vi "Periodic Tasks.vi"(8 "error in":errorcluster) -> ()   [LabVIEW 2015]
doc: "This VI runs in parallel to other tasks. It can contain as many user-defined periodic loops as you need. These can carry out PID or other sorts of timed response."
uses:
  sprocket/src/Refname/Refname Enum (Actuator).ctl
  sprocket/src/Action/Action Name.ctl
  <vilib>/Rock Robotics/SystemInterfaces/Utilities/FPGA_UtilitiesLED Source.ctl
  <vilib>/Rock Robotics/SystemInterfaces/Utilities/FPGA_UtilitiesLED State.ctl
  <vilib>/Rock Robotics/WPI/Compressor/WPI_CompressorGetSetRefNum.vi
  <vilib>/Rock Robotics/WPI/RobotDrive/WPI_RobotDriveGetSetRefNum.vi
  Robot Global Data.vi
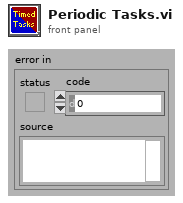
[diagram p1: front panel]
types:
  T1 = typedef "Refname Enum (Actuator).ctl" = enum16{"Drive Motors"}
  T2 = typedef "Action.ctl" = cluster{"Name":T3, "Priority":i32, "Data":variant}
  T3 = typedef "Action Name.ctl" = enum16{"No Action", "Drive Left", "Drive Right"}
  T4 = typedef "FPGA_UtilitiesLED State.ctl" = enum16{"Off", "On", "Toggle"}
  T5 = typedef "FPGA_UtilitiesLED Source.ctl" = enum16{"User LED", "FPGA LED"}
  T6 = typedef "WPI_CompressorDevRef.ctl" = cluster{"DevStatus":errorcluster, "DigitalInputDevRef":T7, "RelayDevRef":T10}
  T7 = typedef "WPI_DigitalInputDevRef.ctl" = cluster{"DevStatus":errorcluster, "DIO Channel":T8, "Digital Module":T9}
  T8 = typedef "FPGA_DIOChannel.ctl" = enum8{"DIO 1", "DIO 2", "DIO 3", "DIO 4", "DIO 5", "DIO 6", "DIO 7", "DIO 8", "DIO 9", "DIO 10", "DIO 11", "DIO 12", "DIO 13", "DIO 14", "Invalid"}
  T9 = typedef "FPGA_TypedefDigitalModule.ctl" = enum16{"Digital Module 1", "Digital Module 2"}
  T10 = typedef "WPI_RelayDevRef.ctl" = cluster{"DevStatus":errorcluster, "Relay Channel":T11, "Digital Module":T9, "Relay Direction":T12}
  T11 = typedef "FPGA_DIORelayChannel.ctl" = enum8{"Relay 1", "Relay 2", "Relay 3", "Relay 4", "Relay 5", "Relay 6", "Relay 7", "Relay 8", "Invalid"}
  T12 = typedef "WPI_RelayDirection.ctl" = enum16{"Both directions", "Forward only", "Reverse only"}
  T13 = typedef "WPI_RobotDriveDevRef.ctl" = cluster{"DevStatus":errorcluster, "Motors[]":T14[], "Square Inputs":bool, "Max Output":dbl}
  T14 = typedef "WPI_MotorControlDeviceRef.ctl" = cluster{"DeviceStatus":errorcluster, "Type":enum16{"PWM", "CAN"}, "PWM":cluster{"Digital Module":T9, "PWM Channel":T15, "DeadBand":T16}, "CAN":cluster{"Device Number":u8, "Control Mode":T17, "Semaphore":T18, "Max Vout":dbl}, "Invert":bool, "TransformRef":T19, "InvTransformRef":T19}
  T15 = typedef "FPGA_DIOPWMChannel.ctl" = enum8{"PWM 1", "PWM 2", "PWM 3", "PWM 4", "PWM 5", "PWM 6", "PWM 7", "PWM 8", "PWM 9", "PWM 10", "Invalid"}
  T16 = typedef "WPI_PWMDeadband.ctl" = cluster{"Name":string, "maxPositivePwm":i32, "minPositivePwm":i32, "centerPwm":i32, "maxNegativePwm":i32, "minNegativePwm":i32, "angularRange":u16}
  T17 = typedef "WPI_CANJaguar_ControlMode.ctl" = enum8{"Percent VBus", "Current", "Speed", "Position", "Voltage"}
  T18 = typedef "Semaphore RefNum" = refnum<k1>
  T19 = typedef "WPI_PWMTransform_ConPane.ctl" = refnum<vi>
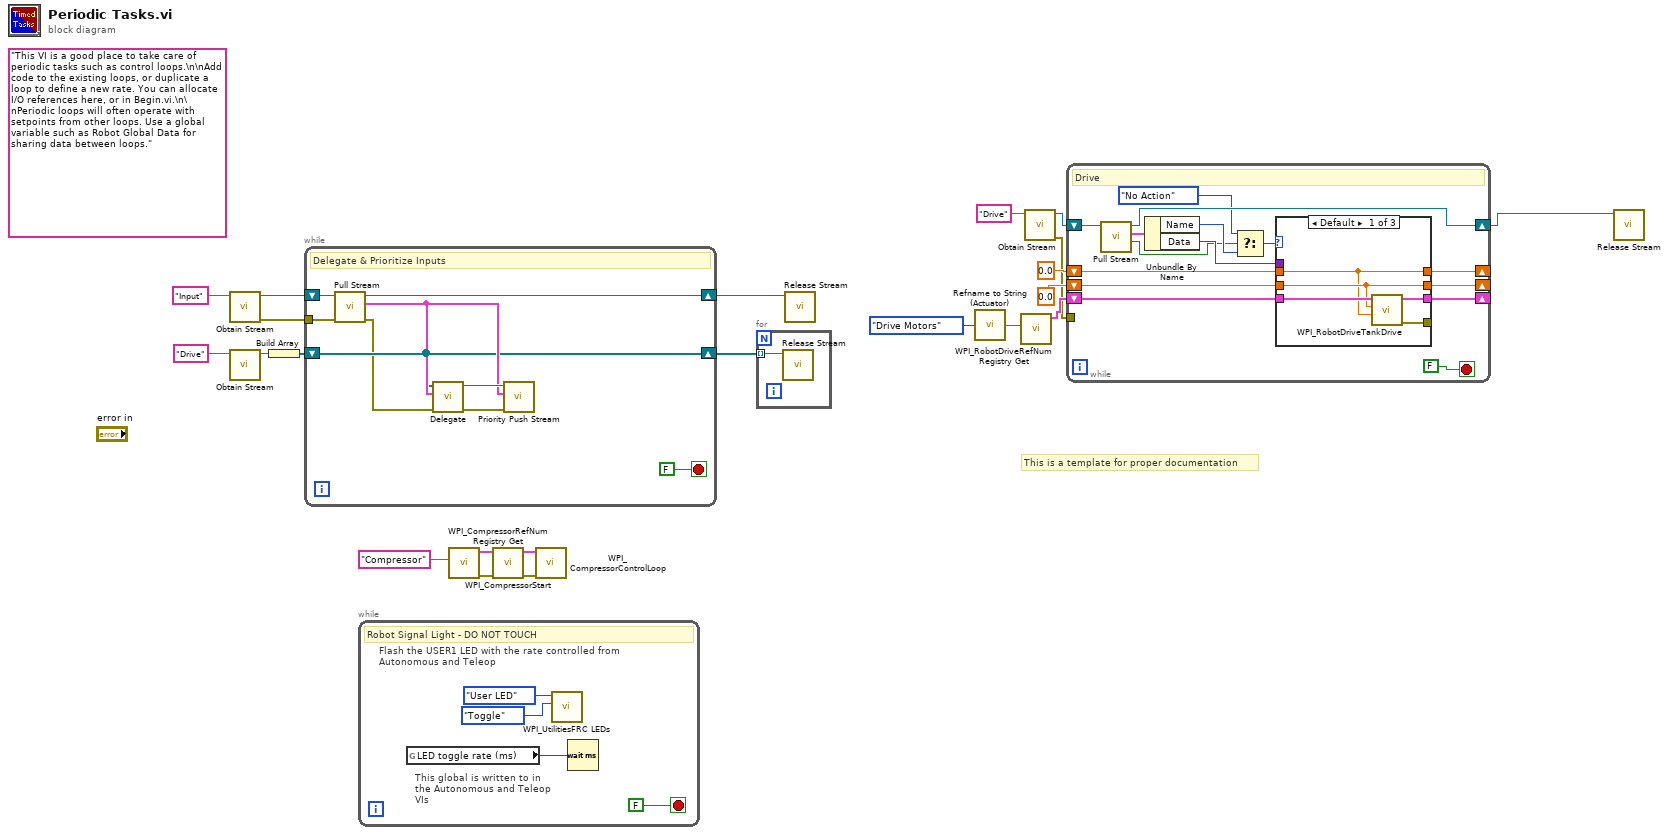
[diagram p0: block diagram]
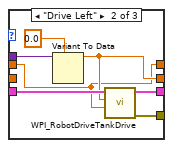
[diagram p2: hidden frame]
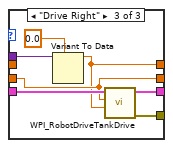
[diagram p3: hidden frame]
diagram:
  (unwired) "This VI is a good place to take care of periodic tasks such as control loops.\n\nAdd code to the existing loops, or duplicate a loop to define a new rate. You can allocate I/O references here, or in Begin.vi.\n\nPeriodic loops will often operate with setpoints from other loops. Use a global variable such as Robot Global Data for sharing data between loops."
  # "This is a template for proper documentation"
  n1 = call "Obtain Stream.vi"("Name"="Input") -> ("error out"=w19:errorcluster, "stream out"=w16:refnum<queue>)  [unwired: 9 in]
  n2 = call "Obtain Stream.vi"("Name"="Drive") -> ("stream out"=w17:refnum<queue>)  [unwired: 9 in, 1 out]
  n3 = Build Array(w17) -> (w18:refnum<queue>[])
  n4 = while {
    shift-right: [w29] -> w21
    shift-left: w16 -> [w30]
    shift-right: [w25] -> w20
    shift-left: w18 -> [w25]
    tunnel: w19 -> [w27]
    stop <- FALSE stop-if-true
    # "Delegate & Prioritize Inputs"
    n5 = call "Pull Stream.vi"("error in (no error)"=w27, "stream in"=w30) -> ("error out"=w24:errorcluster, "element"=w26:T2, "queue out"=w29:refnum<queue>)  [unwired: 6 in, 1 out]
    n6 = call "Delegate.vi"("error in (no error)"=w24, "Action"=w26, "Subsystems"=w25) -> ("error out"=w23:errorcluster, "Delegate"=w28:refnum<queue>)  [unwired: 7 in]
    n7 = call "Priority Push Stream.vi"("error in (no error)"=w23, "Action"=w26, "Subsystem in"=w28) -> ()  [unwired: 7 in, 2 out]
  }
  n8 = while {
    stop <- FALSE stop-if-true
    # "This global is written to in the Autonomous and Teleop VIs"
    # "Flash the USER1 LED with the rate controlled from Autonomous and Teleop"
    # "Robot Signal Light - DO NOT TOUCH"
    n9 = global read "Robot Global Data.vi" "LED toggle rate (ms)"() -> (w32:u32)
    n10 = call <vilib>:"WPI_UtilitiesFRC LEDs.vi"("State"=FPGA_UtilitiesLED_State."Toggle", "LED Type"=FPGA_UtilitiesLED_Source."User LED") -> ()  [unwired: 1 in, 9 out]
    n11 = Wait (ms)(milliseconds to wait=w32) -> ()  [unwired: 1 out]
  }
  n12 = call <vilib>:"WPI_CompressorRefNum Registry Get.vi"("refnum name"="Compressor") -> ("error out"=w3:errorcluster, "CompressorDevRef"=w4:T6)  [unwired: 9 in]
  n13 = call <vilib>:"WPI_CompressorStart.vi"("error in (no error)"=w3, "CompressorDevRef"=w4) -> ("error out"=w2:errorcluster, "CompressorDevRef"=w5:T6)  [unwired: 8 in]
  n14 = call <vilib>:"WPI_CompressorControlLoop.vi"("error in (no error)"=w2, "CompressorDevRef"=w5) -> ()  [unwired: 10 in]
  n15 = for {
    tunnel: w20 -> [w36] mode=indexing
    n16 = call "Release Stream.vi"("stream in"=w36) -> ()  [unwired: 9 in, 2 out]
  }
  n17 = call "Release Stream.vi"("stream in"=w21) -> ()  [unwired: 9 in, 2 out]
  n18 = call "Refname to String (Actuator).vi"("Actuator Refname"=Refname_Enum_(Actuator)."Drive Motors") -> ("Refnum Name"=w9:string)
  n19 = call <vilib>:"WPI_RobotDriveRefNum Registry Get.vi"("refnum name"=w9) -> ("RobotDriveDevRef"=w11:T13)  [unwired: 9 in, 1 out]
  n20 = call "Obtain Stream.vi"("Name"="Drive") -> ("error out"=w1:errorcluster, "stream out"=w7:refnum<queue>)  [unwired: 9 in]
  n21 = while {
    shift-right: [w51] -> w8
    shift-left: w7 -> [w37]
    shift-right: [w42] -> _
    shift-left: w11 -> [w47]
    shift-right: [w45] -> _
    shift-left: 0.0 -> [w44]
    shift-right: [w46] -> _
    shift-left: 0.0 -> [w43]
    tunnel: w1 -> [_]
    stop <- FALSE stop-if-true
    # "Drive"
    n22 = call "Pull Stream.vi"("stream in"=w37) -> ("timed out?"=w39:bool, "element"=w49:T2, "queue out"=w51:refnum<queue>)  [unwired: 7 in, 1 out]
    n23 = Unbundle By Name(w49) -> ("Name"=w40:T3, "Data"=w48:variant)
    n24 = Select(t=Action_Name."No Action" ("Name"), s=w39, f=w40) -> (s? t:f=w41:T3)
    n25 = case shown="Default" w41 {
      tunnel: w48 -> [_ w62 w69]
      tunnel: w47 -> [w56 w61 w68]
      tunnel: [w53 w58 w65] -> w46
      tunnel: [w54 w59 w66] -> w45
      tunnel: w44 -> [w54 _ w66]
      tunnel: w43 -> [w53 w58 _]
      tunnel: [w55 w60 w67] -> w42
      tunnel: [w52 w57 w64] -> _
      frame Default {
        n26 = call <vilib>:"WPI_RobotDriveTankDrive.vi"("Right axis value"=w53, "Left axis value"=w54, "RobotDriveDevRef"=w56) -> ("error out"=w52:errorcluster, "RobotDriveDevRef"=w55:T13)  [unwired: 6 in, 1 out]
      }
      frame "Drive Left" {
        n27 = Variant To Data(type=0.0, Variant=w62) -> (data=w59:dbl)  [unwired: 1 in, 1 out]
        n28 = call <vilib>:"WPI_RobotDriveTankDrive.vi"("Right axis value"=w58, "Left axis value"=w59, "RobotDriveDevRef"=w61) -> ("error out"=w57:errorcluster, "RobotDriveDevRef"=w60:T13)  [unwired: 6 in, 1 out]
      }
      frame "Drive Right" {
        n29 = Variant To Data(type=0.0, Variant=w69) -> (data=w65:dbl)  [unwired: 1 in, 1 out]
        n30 = call <vilib>:"WPI_RobotDriveTankDrive.vi"("Right axis value"=w65, "Left axis value"=w66, "RobotDriveDevRef"=w68) -> ("error out"=w64:errorcluster, "RobotDriveDevRef"=w67:T13)  [unwired: 6 in, 1 out]
      }
    }
  }
  n31 = call "Release Stream.vi"("stream in"=w8) -> ()  [unwired: 9 in, 2 out]
